vi "getMainDescriptor.vi"(8 "error in (no error)":errorcluster, 11 "IMultiReaderStatus in":refnum<class "IMultiReaderStatus.lvclass">) -> (0 "error out":errorcluster, 2 "EventPacket out":refnum<class "IEventPacket.lvclass">, 3 "IMultiReaderStatus out":refnum<class "IMultiReaderStatus.lvclass">)   [LabVIEW 2022 SP3, in "openDAQ.lvlib" / "IBaseObject.lvlib" / "IReaderStatus.lvlib" / "IMultiReaderStatus.lvlib" / "IMultiReaderStatus.lvclass"]
uses:
  <instrlib>/openDAQ/Public/Classes/IMultiReaderStatus/IMultiReaderStatus.lvclass
  C:/Program Files (x86)/National Instruments/LabVIEW 2022/instr.lib/openDAQ/Public/Classes/IBaseObject/IBaseObject.lvclass
  <instrlib>/openDAQ/Public/Classes/IEventPacket/IEventPacket.lvclass
  <instrlib>/openDAQ/Public/Classes/IBaseObject/IBaseObject.lvclass/IBaseObject.ctl
  <instrlib>/openDAQ/Public/Classes/IBaseObject/Accessor/Read reference.vi
  <instrlib>/openDAQ/Public/Classes/IBaseObject/Accessor/Write reference.vi
  <instrlib>/openDAQ/Binaries/Windows/x86/copendaq32.dll
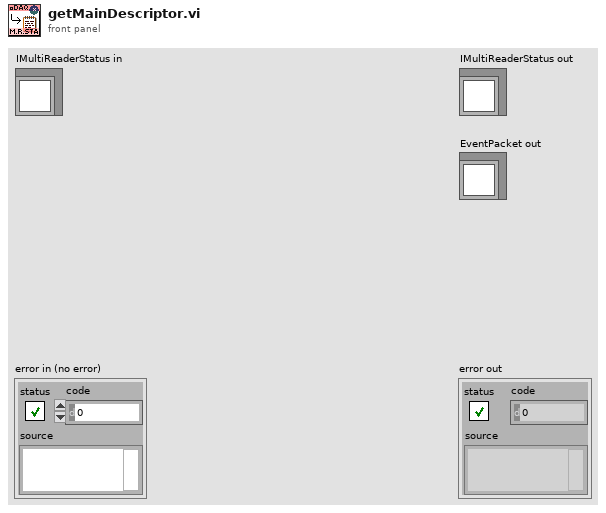
[diagram p1: front panel]
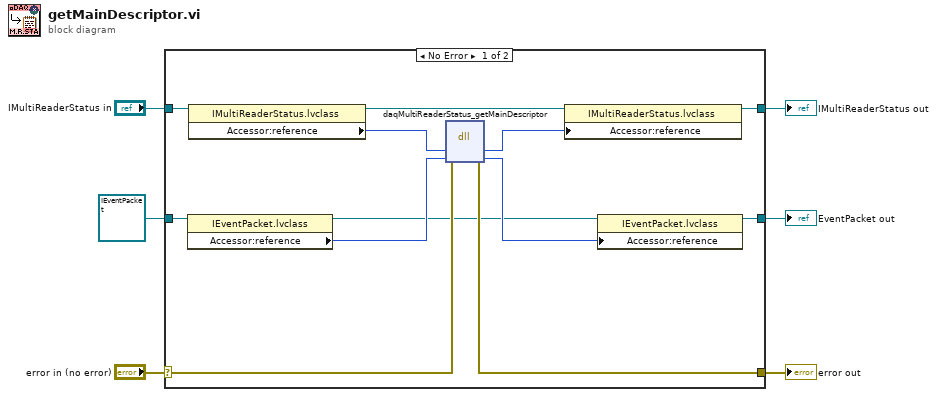
[diagram p0: block diagram]
diagram:
  n1 = case shown="No Error" "error in (no error)" {
    selector: "error in (no error)" -> [w17 w21]
    tunnel: [w16 w21] -> w5
    tunnel: [w14 w20] -> w3
    tunnel: "IMultiReaderStatus in" -> [w18 w20]
    tunnel: refnum<class "IEventPacket.lvclass"> refnum ("openDAQ.lvlib:IBaseObject.lvlib:IPacket.lvlib:IEventPacket.lvlib:IEventPacket.lvclass") -> [w11 w19]
    tunnel: [w7 w19] -> w1
    frame No Error {
      n2 = property class="IEventPacket.lvclass"(reference=w11) -> (reference out=w8:refnum<class "IEventPacket.lvclass">, "Accessor:reference"=w10:i64)  [unwired: 1 in, 1 out]
      n3 = property class="IMultiReaderStatus.lvclass"(reference=w18) -> (reference out=w15:refnum<class "IMultiReaderStatus.lvclass">, "Accessor:reference"=w13:i64)  [unwired: 1 in, 1 out]
      n4 = dll-call lib="C:/Program Files (x86)/National Instruments/LabVIEW 2022/instr.lib/openDAQ/Binaries/Windows/x86/copendaq*.*" fn="daqMultiReaderStatus_getMainDescriptor"(error in=w17, "status"=w13, "descriptor"=w10) -> (error out=w16:errorcluster, "status"=w12:i64, "descriptor"=w9:i64)  [unwired: 3 in, 1 out]
      n5 = property class="IMultiReaderStatus.lvclass"(reference=w15, "Accessor:reference"=w12) -> (reference out=w14:refnum<class "IMultiReaderStatus.lvclass">)  [unwired: 1 in, 1 out]
      n6 = property class="IEventPacket.lvclass"(reference=w8, "Accessor:reference"=w9) -> (reference out=w7:refnum<class "IEventPacket.lvclass">)  [unwired: 1 in, 1 out]
    }
    frame Error {
    }
  }
  "error out" <- w5
  "IMultiReaderStatus out" <- w3
  "EventPacket out" <- w1
